vi "Gui_SetupExcitation.vi"(7 "Variant For Path":variant, 8 "error in (no error)":errorcluster, 10 "Excit Table Variant":variant, 11 "Variant":variant) -> (0 "error out":errorcluster caption="sortie d'erreur", 2 "Excit Table Variant Output":variant, 3 "Variant Output":variant)   [LabVIEW 2018]
doc: "This VI setup the parameters for the excitation waveforms.\n\n1. Init the table of Waveforms with the previous values.\n2. Wait for the user events, CTRL-Z is disabled.\n3. If any cell of the table has changed, start a Check and create a new excit script\n4. When OK is pushed, generate and store the waveforms to disk."
uses:
  controls/EXCIT_Form_Selector.ctl
  controls/EXPERT_Inputs.ctl
  controls/DIGIT_5122_Inputs.ctl
  <instrlib>/niScope/Controls/niScope trigger source.ctl
  controls/HSDIO_6541_Inputs.ctl
  <instrlib>/niHSDIO/niHSDIO.llb/niHSDIO_ctl Trigger Source Values (Ring).ctl
  controls/SOFTWARE_Inputs.ctl
  controls/AO_6711_Inputs.ctl
  controls/AWG_5421_Inputs.ctl
  <instrlib>/niFgen/niFgen.llb/niFgen_ctl Trigger Source Values (Ring).ctl
  controls/XML_Inputs.ctl
  controls/EXCIT_Table.ctl
  controls/SEQUENCE_Inputs.ctl
  controls/EXCIT_Inputs.ctl
  controls/DATA_Inputs.ctl
  controls/TIMING_Inputs.ctl
  controls/PROCESSING_Inputs.ctl
  controls/TRAPPING_Inputs.ctl
panel:
  in  "SEQUENCE Inputs":T1={"EXCIT Inputs"={"Number of Excitations"=1, "Script Text"="", "Table of Waveforms"=[]}, "DATA Inputs"={"Record Length"=524000, "Sample Rate"=2000000.0, "Data Type"=0, "Vertical Range"=10.0, "Acquisition Duration"=262.0}, "TIMING Inputs"={"Number of Acquisitions "=1, "Number of Accumulations"=1, "Table of Waveforms"=[], "Script Text"=""}, "PROCESSING Inputs"={"Reference Mass"=300.0939, "Cyclotron Freq"=255.727, "Magnetron Freq"=0.001}, "TRAPPING Inputs"={"Number of Channels"=4, "Init Values"=[2.0, 9.0, 2.0, 9.0], "Opening Values"=[0.0, 0.0, 0.0, 0.0], "Trapping Values"=[2.0, 9.0, 2.0, 9.0], "Emptying Values"=[-10.0, -10.0, -10.0, -10.0], "Adiabatic ON"=FALSE, "Adiabatic Duration"=100, "Adiabatic Waveforms"=["Adiabatic_None_2_2_2000", "Adiabatic_Ramp_9_0_2000", "Adiabatic_None_2_2_2000", "Adiabatic_RC_9_0_2000"], "Ions Refill ON"=FALSE, "Number of Ions Refills"=1, "Trapping Delay"=400.0, "Trapping Duration"=300.0}} {"TRAPPING Inputs"."Trapping Duration" min=2.0; "TRAPPING Inputs"."Trapping Delay" min=2.0; "TRAPPING Inputs"."Number of Ions Refills" min=1 max=1000; "TRAPPING Inputs"."Trapping Values" min=-10.0 max=10.0; "TRAPPING Inputs"."Init Values" min=-10.0 max=10.0; "TRAPPING Inputs"."Emptying Values" min=-10.0 max=10.0; "TRAPPING Inputs"."Opening Values" min=-10.0 max=10.0; "PROCESSING Inputs"."Magnetron Freq" format="%.5g"; "PROCESSING Inputs"."Cyclotron Freq" format="%.5g"; "PROCESSING Inputs"."Reference Mass" format="%.5g"; "TIMING Inputs"."Number of Accumulations" min=0 max=50 step=1; "TIMING Inputs"."Number of Acquisitions" min=1 max=10 step=1; "DATA Inputs"."Vertical Range" items=["0.2"=0.2, "0.4"=0.4, "1"=1.0, "2"=2.0, "4"=4.0, "10"=10.0]; "DATA Inputs"."Data Type" items=["I16", "DBL"]; "DATA Inputs"."Sample Rate" items=["1 MHz"=1000000.0, "2 MHz"=2000000.0, "5 MHz"=5000000.0, "10 MHz"=10000000.0, "20 MHz"=20000000.0, "25 MHz"=25000000.0, "50 MHz"=50000000.0, "100 MHz"=100000000.0]; "EXCIT Inputs"."Number of Excitations" min=1 max=10}
  in  "EXCIT Table":T7={"Number of Excits"=0, "Number of Ejects"=0, "Sampling Frequency"=0.0, "Waveforms Table"=[["Excit1", "name", "Swift", "0.5", "1200", "70", "150", "550", "0", "0", "0"]]}
  in  "EXPERT Inputs":T8={"DIGIT 5122 Inputs"={"Sample Rate"=1.0, "Resource Name"="Digitizer", "Channel Name"="0", "Trigger Source"="VAL_EXTERNAL", "Vertical Range"=10.0, "Trigger Level"=3.0}, "HSDIO 6541 Inputs"={"Resource Name"="SequencerHSDIO", "Clock Rate"=1000000.0, "Trigger Source"="PFI0"}, "SOFTWARE Inputs"={"Application Directory"=path "D:/S.O.F.T.S/LABVIEW/PIL", "Software Version"="1.0.0", "Data Path"=path "D:/PIRENEA/DATA", "XML Path"=path "D:/PIRENEA/DATA", "XML File Filter"="*.xml", "XML Saved Path"=path "D:/PIRENEA/DATA", "Excit Scripts Path"=path "D:/PIRENEA/EXCIT_SCRIPTS", "Excit Scripts File Filter"="*.txt", "Excit Waveforms Path"=path "D:/PIRENEA/EXCIT_WFMS", "Excit Waveforms File Filter"="*.bin", "Timing Scripts Path"=path "D:/PIRENEA/SEQUENCE_SCRIPTS", "Timing Scripts File Filter"="*.txt", "Timing Waveforms Path"=path "D:/PIRENEA/SEQUENCE_WFMS", "Timing Waveforms File Filter"="*.bin", "Trapping Waveforms Path"=path "D:/PIRENEA/TRAPPING_WFMS", "Trapping Waveforms File Filter"="*.bin"}, "AO 6711 Inputs"={"Physical Channels"="AnalogOutput/ao0:3", "Min Voltage"=-10.0, "Max Voltage"=10.0, "Trigger Source"="/AnalogOutput/PFI0", "Counter"="AnalogOutput/ctr0"}, "AWG 5421 Inputs"={"Resource Name"="WaveformGenerator", "Sample Rate"=0.0, "Trigger Type"=4, "Trigger Source"="PFI0", "Waveform Gain"=0.31, "Digital Filter ON"=TRUE}, "XML Inputs"={"Version Tag Name"="XML_Version", "Version String"="1.0"}} {"AWG 5421 Inputs"."Sample Rate" format="%.2p"; "AWG 5421 Inputs"."Trigger Type" items=["None", "Software Edge", "Digital Edge", "Digital Level"]; "AO 6711 Inputs"."Max Voltage" min=-10.0 max=10.0; "AO 6711 Inputs"."Min Voltage" min=-10.0 max=10.0; "HSDIO 6541 Inputs"."Clock Rate" format="%.2p"; "DIGIT 5122 Inputs"."Trigger Level" format="%.2f"; "DIGIT 5122 Inputs"."Vertical Range" format="%.2f"; "DIGIT 5122 Inputs"."Sample Rate" step=65535.0 format="%#_3p"}
  in  "CANCEL":bool
  in  "Sampling Frequency":dbl(ring)=10.0 caption="Sampling (MHz)" items=["10"=10.0, "20"=20.0, "25"=25.0, "50"=50.0, "100"=100.0]
  out "Excitation FFT":cluster{dbl[], "Power Spectrum (V^2 rms)":dbl[]}(graph)
  in  "Graph ID":i32
  out "Excitation Signal":T18(graph)
  in  "Excit Form":T19
  in  "CHECK":bool
  in  "Waveforms Table":i32(listbox)
  out "Number of Ejects":u16=1
  out "Number of Excits":u16=3
  out "Script Text":string
  in  "OK":bool
  # "GO_out"
  # "Gout"
  # "GI_in"
  # "Gin"
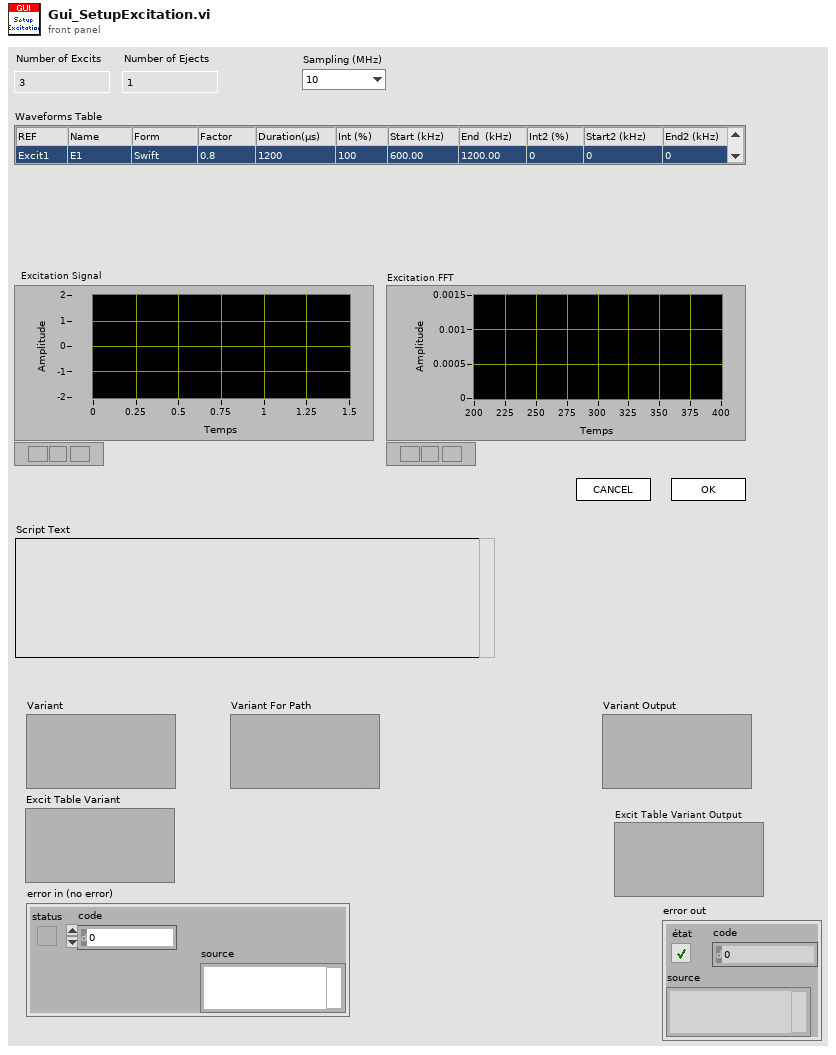
[diagram p1: front panel]
types:
  T1 = typedef "SEQUENCE_Inputs.ctl" = cluster{"EXCIT Inputs":T2, "DATA Inputs":T3, "TIMING Inputs":T4, "PROCESSING Inputs":T5, "TRAPPING Inputs":T6}
  T2 = typedef "EXCIT_Inputs.ctl" = cluster{"Number of Excitations":i32, "Script Text":string, "Table of Waveforms":string[]}
  T3 = typedef "DATA_Inputs.ctl" = cluster{"Record Length":i32, "Sample Rate":dbl, "Data Type":u8, "Vertical Range":dbl, "Acquisition Duration":dbl}
  T4 = typedef "TIMING_Inputs.ctl" = cluster{"Number of Acquisitions ":i16, "Number of Accumulations":i16, "Table of Waveforms":string[], "Script Text":string}
  T5 = typedef "PROCESSING_Inputs.ctl" = cluster{"Reference Mass":dbl, "Cyclotron Freq":dbl, "Magnetron Freq":dbl}
  T6 = typedef "TRAPPING_Inputs.ctl" = cluster{"Number of Channels":i32, "Init Values":dbl[], "Opening Values":dbl[], "Trapping Values":dbl[], "Emptying Values":dbl[], "Adiabatic ON":bool, "Adiabatic Duration":i32, "Adiabatic Waveforms":string[], "Ions Refill ON":bool, "Number of Ions Refills":i32, "Trapping Delay":dbl, "Trapping Duration":dbl}
  T7 = typedef "EXCIT_Table.ctl" = cluster{"Number of Excits":u16, "Number of Ejects":u16, "Sampling Frequency":dbl, "Waveforms Table":string[][]}
  T8 = typedef "EXPERT_Inputs.ctl" = cluster{"DIGIT 5122 Inputs":T9, "HSDIO 6541 Inputs":T11, "SOFTWARE Inputs":T13, "AO 6711 Inputs":T14, "AWG 5421 Inputs":T15, "XML Inputs":T17}
  T9 = typedef "DIGIT_5122_Inputs.ctl" = cluster{"Sample Rate":dbl, "Resource Name":refnum<k15>, "Channel Name":string, "Trigger Source":T10, "Vertical Range":dbl, "Trigger Level":dbl}
  T10 = typedef "niScope trigger source.ctl" = string
  T11 = typedef "HSDIO_6541_Inputs.ctl" = cluster{"Resource Name":refnum<k15>, "Clock Rate":dbl, "Trigger Source":T12}
  T12 = typedef "niHSDIO_ctl Trigger Source Values (Ring).ctl" = string
  T13 = typedef "SOFTWARE_Inputs.ctl" = cluster{"Application Directory":path, "Software Version":string, "Data Path":path, "XML Path":path, "XML File Filter":string, "XML Saved Path":path, "Excit Scripts Path":path, "Excit Scripts File Filter":string, "Excit Waveforms Path":path, "Excit Waveforms File Filter":string, "Timing Scripts Path":path, "Timing Scripts File Filter":string, "Timing Waveforms Path":path, "Timing Waveforms File Filter":string, "Trapping Waveforms Path":path, "Trapping Waveforms File Filter":string}
  T14 = typedef "AO_6711_Inputs.ctl" = cluster{"Physical Channels":tag, "Min Voltage":dbl, "Max Voltage":dbl, "Trigger Source":tag, "Counter":tag}
  T15 = typedef "AWG_5421_Inputs.ctl" = cluster{"Resource Name":refnum<k15>, "Sample Rate":dbl, "Trigger Type":u16, "Trigger Source":T16, "Waveform Gain":dbl, "Digital Filter ON":bool}
  T16 = typedef "niFgen_ctl Trigger Source Values (Ring).ctl" = string
  T17 = typedef "XML_Inputs.ctl" = cluster{"Version Tag Name":string, "Version String":string}
  T18 = cluster{"X Time":dbl[], "Signal Excitation":dbl[]}
  T19 = typedef "EXCIT_Form_Selector.ctl" = enum16{"Swift", "TwoSwift", "Chirp", "Sinus", "Ramp"}
  T20 = typedef "LVPoint32TypeDef.ctl" = cluster{"Horizontal":i32, "Vertical":i32}
  T21 = typedef "LVRowAndColumnTypeDef.ctl" = cluster{"Row":i32, "Column":i32}
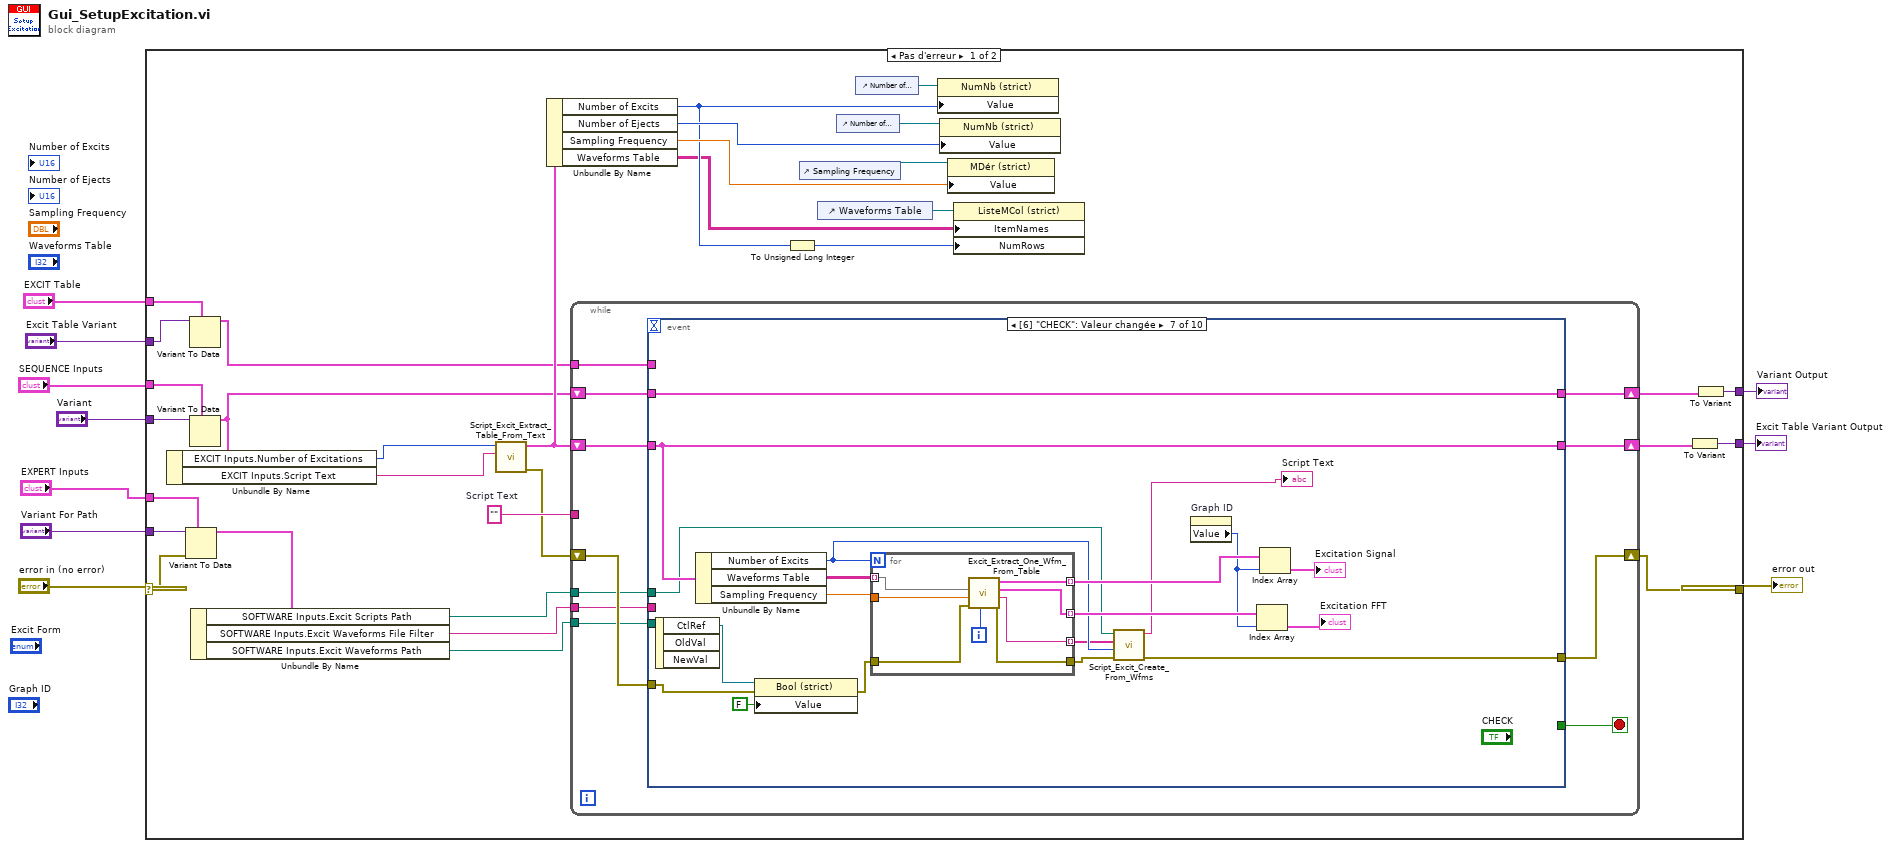
[diagram p0: block diagram]
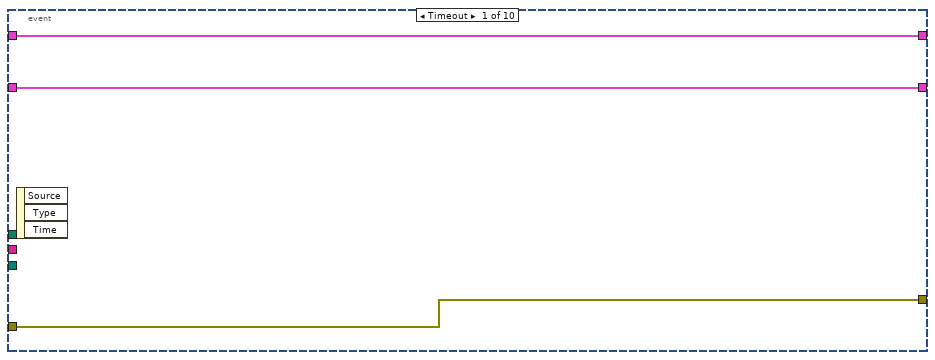
[diagram p2: hidden frame]
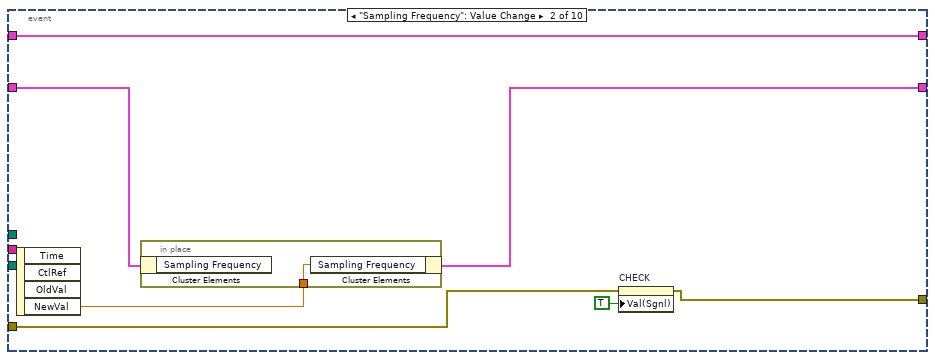
[diagram p3: hidden frame]
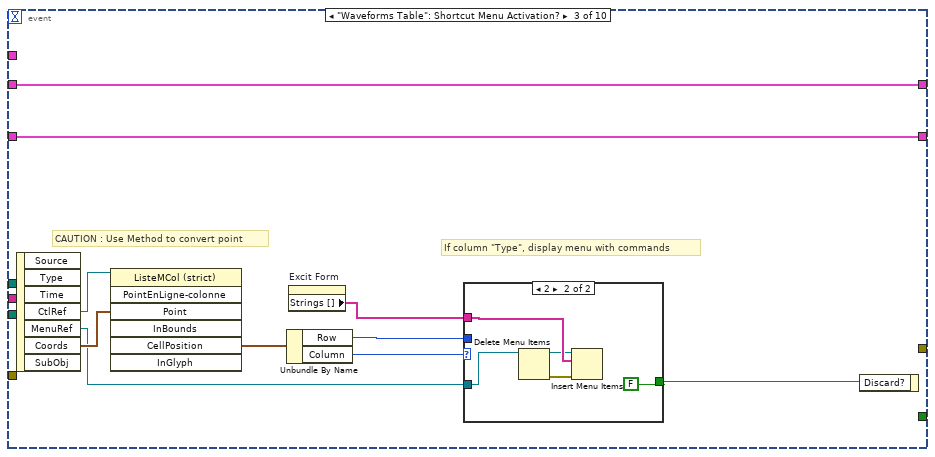
[diagram p4: hidden frame]
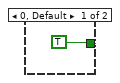
[diagram p5: hidden frame]
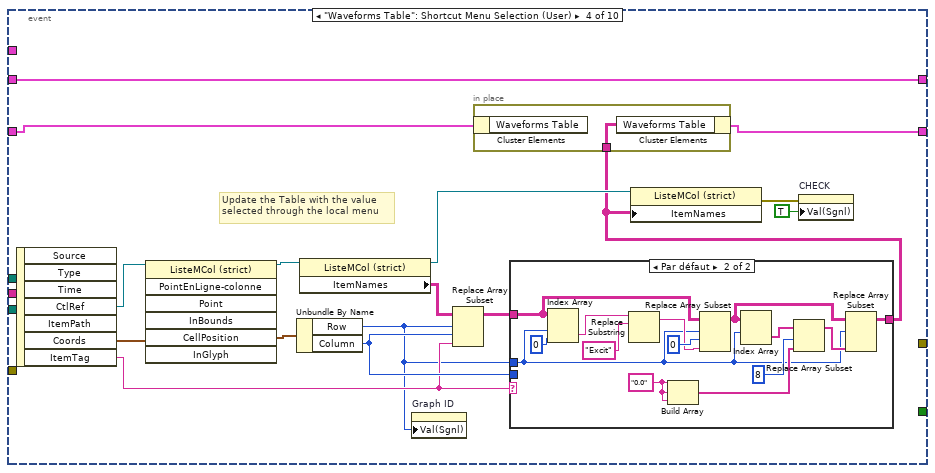
[diagram p6: hidden frame]
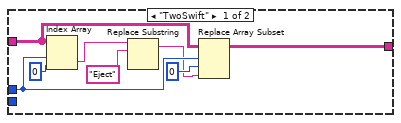
[diagram p7: hidden frame]
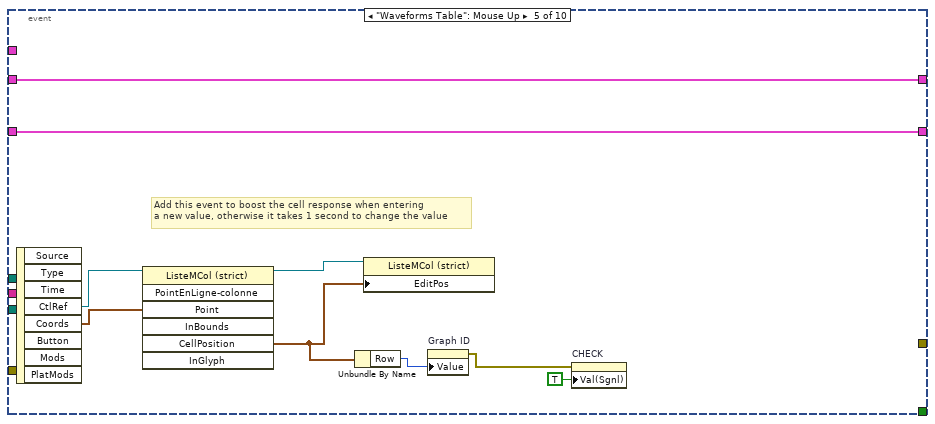
[diagram p8: hidden frame]
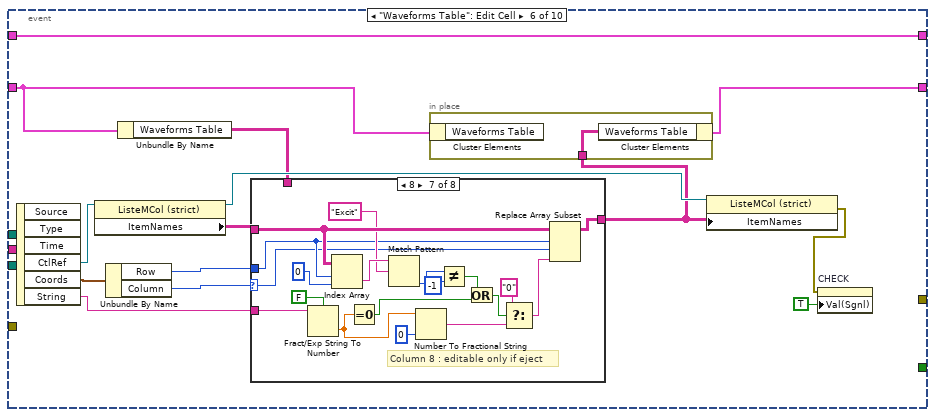
[diagram p9: hidden frame]
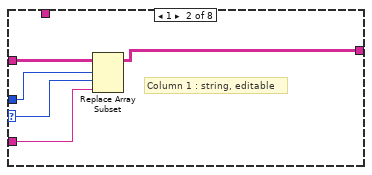
[diagram p11: hidden frame]
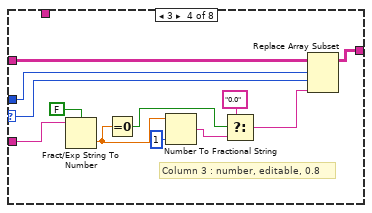
[diagram p13: hidden frame]
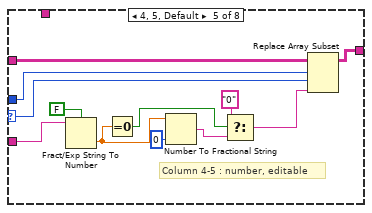
[diagram p14: hidden frame]
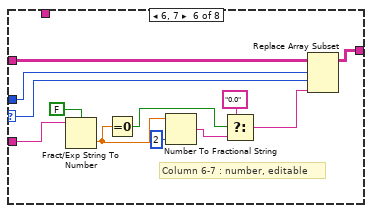
[diagram p15: hidden frame]
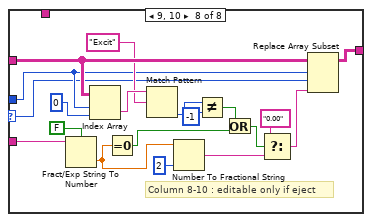
[diagram p16: hidden frame]
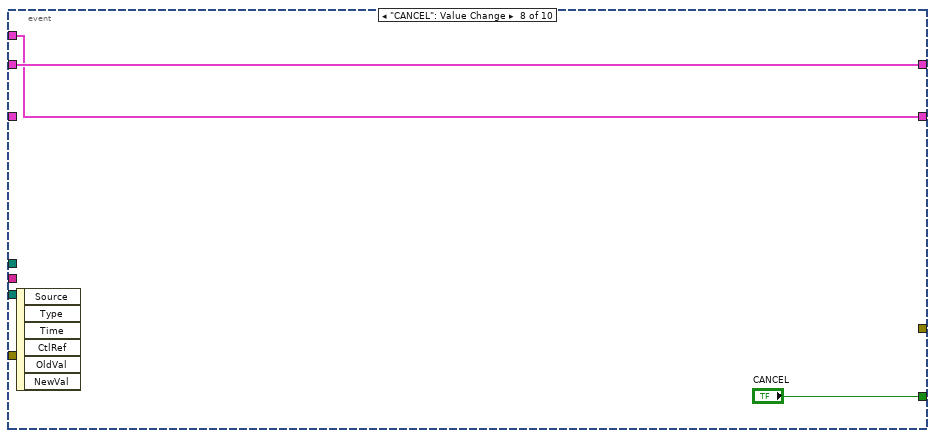
[diagram p17: hidden frame]
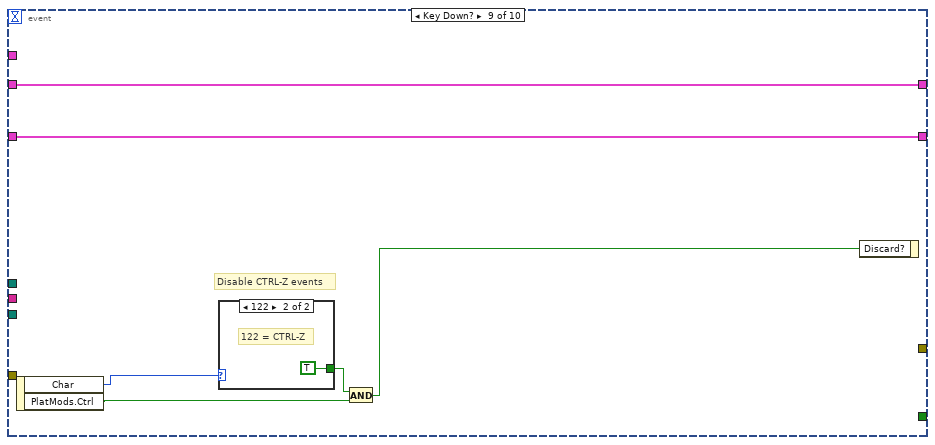
[diagram p18: hidden frame]
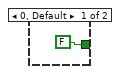
[diagram p19: hidden frame]
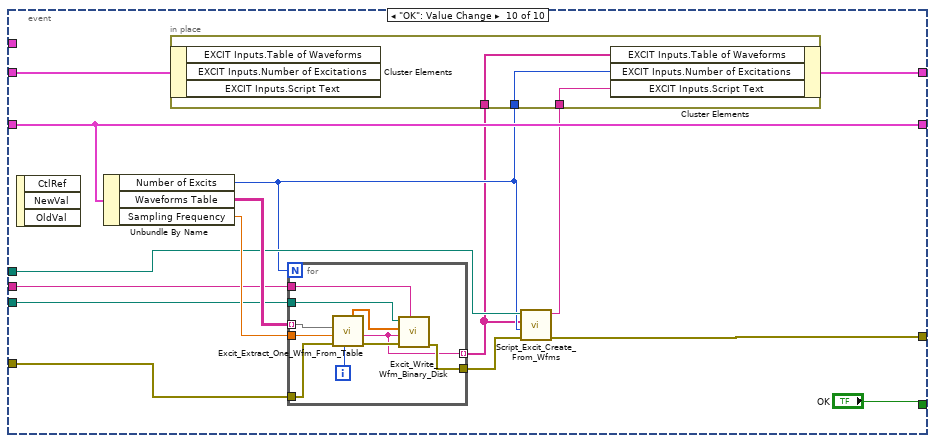
[diagram p20: hidden frame]
diagram:
  n1 = case shown="Pas d'erreur" "error in (no error)" {
    selector: "error in (no error)" -> [w38 w293]
    tunnel: [w26 w293] -> w9
    tunnel: "Variant" -> [w40 w292]
    tunnel: "Variant For Path" -> [w41 _]
    tunnel: [w39 w292] -> w6
    tunnel: [w17 w291] -> w4
    tunnel: "Excit Table Variant" -> [w16 w291]
    tunnel: "EXPERT Inputs" -> [w13 _]
    tunnel: "EXCIT Table" -> [w12 _]
    tunnel: "SEQUENCE Inputs" -> [w11 _]
    frame No Error {
      w31 = ""  # Script Text
      n2 = Variant To Data(error in=w38, type=w13, Variant=w41) -> (data=w42:T8)  [unwired: 1 out]
      n3 = Variant To Data(type=w12, Variant=w16) -> (data=w15:T7)  [unwired: 1 in, 1 out]
      n4 = Variant To Data(type=w11, Variant=w40) -> (data=w24:T1)  [unwired: 1 in, 1 out]
      n5 = Unbundle By Name(w24) -> ("EXCIT Inputs.Number of Excitations"=w14:i32, "EXCIT Inputs.Script Text"=w19:string)
      n6 = Unbundle By Name(w42) -> ("SOFTWARE Inputs.Excit Scripts Path"=w20:path, "SOFTWARE Inputs.Excit Waveforms File Filter"=w21:string, "SOFTWARE Inputs.Excit Waveforms Path"=w22:path)
      n7 = call "Script_Excit_Extract_Table_From_Text.vi"("Excit Text"=w19, "Number of Excitations"=w14) -> ("error out"=w27:errorcluster, "EXCIT Table"=w29:T7)  [unwired: 7 in, 1 out]
      n8 = Unbundle By Name(w29) -> ("Number of Excits"=w32:u16, "Number of Ejects"=w35:u16, "Sampling Frequency"=w34:dbl, "Waveforms Table"=w30:string[][])
      n9 = while {
        shift-right: [w49] -> w26
        shift-left: w27 -> [w53]
        shift-right: [w50] -> w18
        shift-left: w29 -> [w52]
        tunnel: w31 -> [_]
        shift-right: [w47] -> w25
        shift-left: w24 -> [w48]
        tunnel: w22 -> [w46]
        tunnel: w21 -> [w45]
        tunnel: w20 -> [w44]
        tunnel: w15 -> [w43]
        stop <- w51 stop-if-true
        n10 = event shown="[6] \"CHECK\": Valeur changée" {
          selector: _ -> [_ _ _ _ _ _ _ _ _ _]
          dyn-events: _ -> [_ _ _ _ _ _ _ _ _ _]
          timeout: _ -> [_ _ _ _ _ _ _ _ _ _]
          tunnel: w53 -> [w55 w57 _ _ _ _ w226 _ _ w273]
          tunnel: w52 -> [w56 w63 w67 w90 w126 w137 w243 _ w255 w274]
          tunnel: [w56 w61 w67 w89 w126 w133 w243 w252 w255 w274] -> w50
          tunnel: [_ _ _ _ _ _ _ "CANCEL" _ "OK"] -> w51
          tunnel: [w55 w58 _ _ _ _ w235 _ _ w266] -> w49
          tunnel: w48 -> [w54 w60 w65 w88 w125 w132 w234 w254 w260 w270]
          tunnel: [w54 w60 w65 w88 w125 w132 w234 w254 w260 w269] -> w47
          tunnel: w46 -> [_ _ _ _ _ _ _ _ _ w272]
          tunnel: w45 -> [_ _ _ _ _ _ _ _ _ w271]
          tunnel: w44 -> [_ _ _ _ _ _ w225 _ _ w267]
          tunnel: w43 -> [_ _ _ _ _ _ _ w252 _ _]
          event Timeout {
            n11 = event-data() -> ()  [unwired: 1 in, 3 out]
          }
          event "Sampling Frequency": Value Change {
            n12 = event-data() -> ("NewVal"=w62:dbl)  [unwired: 1 in, 3 out]
            n13 = in-place {
              in-place-border: w62 -> [w64]
              n14 = in-place-cluster #1(w63) -> ()  [unwired: 1 out]
              n15 = in-place-cluster #1("Sampling Frequency"=w64) -> (w61:T7)
            }
            n16 = property on="CHECK" class="Bool (strict)"(error in=w57, "Val(Sgnl)"=TRUE ("Valeur (Signalisation)")) -> (error out=w58:errorcluster)  [unwired: 1 in, 1 out]
          }
          event "Waveforms Table": Shortcut Menu Activation? {
            # "If column \"Type\", display menu with commands"
            # "CAUTION : Use Method to convert point"
            n17 = event-data() -> ("CtlRef"=w70:refnum<vi>, "MenuRef"=w69:refnum<k9>, "Coords"=w72:T20)  [unwired: 1 in, 4 out]
            n18 = invoke on="Nœud de méthode" class="ListeMCol (strict)" method="PointEnLigne-colonne"(reference=w70, "Point"=w72) -> ("CellPosition"=w71:T21)  [unwired: 5 in, 6 out]
            n19 = Unbundle By Name(w71) -> ("Row"=w73:i32, "Column"=w74:i32)
            n20 = property on="Excit Form" class="Énum (strict)"() -> ("Strings []"=w66:string[])  [unwired: 2 in, 2 out]
            n21 = case shown="2" w74 {
              tunnel: [TRUE FALSE] -> w68
              tunnel: w73 -> [_ _]
              tunnel: w66 -> [_ w79]
              tunnel: w69 -> [_ w76]
              frame 0, Default {
              }
              frame 2 {
                n22 = Delete Menu Items(9:w76) -> (0:w78:errorcluster, 3:w77:refnum<k9>)  [unwired: 3 in]
                n23 = Insert Menu Items(6:w78, 8:w79, 9:w77) -> ()  [unwired: 3 in, 3 out]
              }
            }
            n24 = event-data("Discard?"=w68) -> ()  [unwired: 1 in, 1 out]
          }
          event "Waveforms Table": Shortcut Menu Selection (User) {
            # "Update the Table with the value\nselected through the local menu"
            n25 = event-data() -> ("CtlRef"=w92:refnum<vi>, "Coords"=w91:T20, "ItemTag"=w85:string)  [unwired: 1 in, 4 out]
            n26 = invoke class="ListeMCol (strict)" method="PointEnLigne-colonne"(reference=w92, "Point"=w91) -> (reference out=w95:refnum<vi>, "CellPosition"=w96:T21)  [unwired: 5 in, 5 out]
            n27 = Unbundle By Name(w96) -> ("Row"=w84:i32, "Column"=w87:i32)
            n28 = property class="ListeMCol (strict)"(reference=w95) -> (reference out=w94:refnum<vi>, "ItemNames"=w93:string[][])  [unwired: 1 in, 1 out]
            n29 = property on="Graph ID" class="NumNb (strict)"("Val(Sgnl)"=w84) -> ()  [unwired: 2 in, 2 out]
            n30 = Replace Array Subset(array=w93, new element=w85, index (row)=w84, index (col)=w87) -> (w86:string[][])
            n31 = case shown="Par défaut" w85 {
              tunnel: w84 -> [w100 w106]
              tunnel: w87 -> [_ _]
              tunnel: w86 -> [w101 w115]
              tunnel: [w97 w105] -> w83
              frame "TwoSwift" {
                n32 = Index Array(array=w101, index (row)=w100, index (col)=0 ("indice désactivé (col)")) -> (element=w103:string)
                n33 = Replace Substring(4:"Eject" ("sous-chaîne (\"\")"), 5:w103) -> (1:w98:string)  [unwired: 2 in, 1 out]
                n34 = Replace Array Subset(array=w101, new element=w98, index (row)=w100, index (col)=0 ("indice désactivé (col)")) -> (w97:string[][])
              }
              frame Default {
                w112 = "0.0" ("nouvel élément/sous-tableau")
                n35 = Index Array(array=w115, index (row)=w106, index (col)=0 ("indice désactivé (col)")) -> (element=w117:string)
                n36 = Replace Substring(4:"Excit" ("sous-chaîne (\"\")"), 5:w117) -> (1:w113:string)  [unwired: 2 in, 1 out]
                n37 = Build Array(w112, w112, w112) -> (w111:string[])
                n38 = Replace Array Subset(array=w115, new element=w113, index (row)=w106, index (col)=0 ("indice désactivé (col)")) -> (w108:string[][])
                n39 = Index Array(array=w108, index (row)=w106) -> (element=w110:string[])  [unwired: 1 in]
                n40 = Replace Array Subset(array=w110, new element=w111, index=8 ("indice désactivé (col)")) -> (w107:string[])
                n41 = Replace Array Subset(array=w108, new element=w107, index (row)=w106) -> (w105:string[][])  [unwired: 1 in]
              }
            }
            n42 = in-place {
              in-place-border: w83 -> [w119]
              n43 = in-place-cluster #2(w90) -> ()  [unwired: 1 out]
              n44 = in-place-cluster #2("Waveforms Table"=w119) -> (w89:T7)
            }
            n45 = property class="ListeMCol (strict)"(reference=w94, "ItemNames"=w83) -> (error out=w82:errorcluster)  [unwired: 1 in, 1 out]
            n46 = property on="CHECK" class="Bool (strict)"(error in=w82, "Val(Sgnl)"=TRUE ("Valeur (Signalisation)")) -> ()  [unwired: 1 in, 2 out]
          }
          event "Waveforms Table": Mouse Up {
            # "Add this event to boost the cell response when entering\na new value, otherwise it takes 1 second to change the value"
            n47 = event-data() -> ("CtlRef"=w127:refnum<vi>, "Coords"=w124:T20)  [unwired: 1 in, 6 out]
            n48 = invoke class="ListeMCol (strict)" method="PointEnLigne-colonne"(reference=w127, "Point"=w124) -> (reference out=w128:refnum<vi>, "CellPosition"=w123:T21)  [unwired: 5 in, 5 out]
            n49 = Unbundle By Name(w123) -> ("Row"=w122:i32)
            n50 = property class="ListeMCol (strict)"(reference=w128, "EditPos"=w123) -> ()  [unwired: 1 in, 2 out]
            n51 = property on="Graph ID" class="NumNb (strict)"("Value"=w122) -> (error out=w121:errorcluster)  [unwired: 2 in, 1 out]
            n52 = property on="CHECK" class="Bool (strict)"(error in=w121, "Val(Sgnl)"=TRUE ("Valeur (Signalisation)")) -> ()  [unwired: 1 in, 2 out]
          }
          event "Waveforms Table": Edit Cell {
            n53 = event-data() -> ("CtlRef"=w134:refnum<vi>, "Coords"=w136:T21, "String"=w135:string)  [unwired: 1 in, 3 out]
            n54 = property class="ListeMCol (strict)"(reference=w134) -> (reference out=w140:refnum<vi>, "ItemNames"=w142:string[][])  [unwired: 1 in, 1 out]
            n55 = Unbundle By Name(w136) -> ("Row"=w131:i32, "Column"=w141:i32)
            n56 = Unbundle By Name(w137) -> ("Waveforms Table"=w139:string[][])
            n57 = case shown="8" w141 {
              selector: w141 -> [_ w145 _ w151 w163 w175 w187 w206]
              tunnel: w135 -> [_ w149 _ w162 w174 w186 w205 w224]
              tunnel: w142 -> [_ w147 _ w153 w165 w177 w197 w216]
              tunnel: w131 -> [_ w146 _ w152 w164 w176 w188 w207]
              tunnel: [w144 w148 w150 w161 w173 w185 w204 w223] -> w138
              tunnel: w139 -> [w144 _ w150 _ _ _ _ _]
              frame 0 {
                # "Column 0 : not editable"
              }
              frame 1 {
                # "Column 1 : string, editable"
                n58 = Replace Array Subset(array=w147, new element=w149, index (row)=w146, index (col)=w145) -> (w148:string[][])
              }
              frame 2 {
                # "Column 2 : choice into a menu"
              }
              frame 3 {
                # "Column 3 : number, editable, 0.8"
                n59 = Fract/Exp String To Number(use system decimal point (T)=FALSE ("utiliser le séparateur décimal du système (V)"), string=w162) -> (number=w157:dbl)  [unwired: 2 in, 1 out]
                n60 = Equal To 0?(x=w157) -> (x = 0?=w154:bool)
                n61 = Number To Fractional String(number=w157, precision (6)=i16 1 ("précision (6)")) -> (F-format string=w155:string)  [unwired: 2 in]
                n62 = Select(t="0.0", s=w154, f=w155) -> (s? t:f=w159:string)
                n63 = Replace Array Subset(array=w153, new element=w159, index (row)=w152, index (col)=w151) -> (w161:string[][])
              }
              frame 4, 5, Default {
                # "Column 4-5 : number, editable"
                n64 = Fract/Exp String To Number(use system decimal point (T)=FALSE ("utiliser le séparateur décimal du système (V)"), string=w174) -> (number=w169:dbl)  [unwired: 2 in, 1 out]
                n65 = Equal To 0?(x=w169) -> (x = 0?=w166:bool)
                n66 = Number To Fractional String(number=w169, precision (6)=i16 0 ("précision (6)")) -> (F-format string=w167:string)  [unwired: 2 in]
                n67 = Select(t="0", s=w166, f=w167) -> (s? t:f=w171:string)
                n68 = Replace Array Subset(array=w165, new element=w171, index (row)=w164, index (col)=w163) -> (w173:string[][])
              }
              frame 6, 7 {
                # "Column 6-7 : number, editable"
                n69 = Fract/Exp String To Number(use system decimal point (T)=FALSE ("utiliser le séparateur décimal du système (V)"), string=w186) -> (number=w181:dbl)  [unwired: 2 in, 1 out]
                n70 = Equal To 0?(x=w181) -> (x = 0?=w178:bool)
                n71 = Number To Fractional String(number=w181, precision (6)=i16 2 ("précision (6)")) -> (F-format string=w179:string)  [unwired: 2 in]
                n72 = Select(t="0.0", s=w178, f=w179) -> (s? t:f=w183:string)
                n73 = Replace Array Subset(array=w177, new element=w183, index (row)=w176, index (col)=w175) -> (w185:string[][])
              }
              frame 8 {
                # "Column 8 : editable only if eject"
                n74 = Fract/Exp String To Number(use system decimal point (T)=FALSE ("utiliser le séparateur décimal du système (V)"), string=w205) -> (number=w200:dbl)  [unwired: 2 in, 1 out]
                n75 = Index Array(array=w197, index (row)=w188, index (col)=0 ("indice désactivé (col)")) -> (element=w195:string)
                n76 = Equal To 0?(x=w200) -> (x = 0?=w192:bool)
                n77 = Match Pattern(string=w195, regular expression="Excit" ("expression régulière")) -> (offset past match=w191:i32)  [unwired: 1 in, 3 out]
                n78 = Number To Fractional String(number=w200, precision (6)=i16 0 ("précision (6)")) -> (F-format string=w198:string)  [unwired: 2 in]
                n79 = Not Equal?(x=w191, y=-1) -> (x != y?=w189:bool)
                n80 = Or(x=w189, y=w192) -> (x .or. y?=w193:bool)
                n81 = Select(t="0", s=w193, f=w198) -> (s? t:f=w202:string)
                n82 = Replace Array Subset(array=w197, new element=w202, index (row)=w188, index (col)=w187) -> (w204:string[][])
              }
              frame 9, 10 {
                # "Column 8-10 : editable only if eject"
                n83 = Fract/Exp String To Number(use system decimal point (T)=FALSE ("utiliser le séparateur décimal du système (V)"), string=w224) -> (number=w219:dbl)  [unwired: 2 in, 1 out]
                n84 = Index Array(array=w216, index (row)=w207, index (col)=0 ("indice désactivé (col)")) -> (element=w214:string)
                n85 = Equal To 0?(x=w219) -> (x = 0?=w211:bool)
                n86 = Match Pattern(string=w214, regular expression="Excit" ("expression régulière")) -> (offset past match=w210:i32)  [unwired: 1 in, 3 out]
                n87 = Number To Fractional String(number=w219, precision (6)=i16 2 ("précision (6)")) -> (F-format string=w217:string)  [unwired: 2 in]
                n88 = Not Equal?(x=w210, y=-1) -> (x != y?=w208:bool)
                n89 = Or(x=w208, y=w211) -> (x .or. y?=w212:bool)
                n90 = Select(t="0.00", s=w212, f=w217) -> (s? t:f=w221:string)
                n91 = Replace Array Subset(array=w216, new element=w221, index (row)=w207, index (col)=w206) -> (w223:string[][])
              }
            }
            n92 = in-place {
              in-place-border: w138 -> [w143]
              n93 = in-place-cluster #3(w137) -> ()  [unwired: 1 out]
              n94 = in-place-cluster #3("Waveforms Table"=w143) -> (w133:T7)
            }
            n95 = property class="ListeMCol (strict)"(reference=w140, "ItemNames"=w138) -> (error out=w130:errorcluster)  [unwired: 1 in, 1 out]
            n96 = property on="CHECK" class="Bool (strict)"(error in=w130, "Val(Sgnl)"=TRUE ("Valeur (Signalisation)")) -> ()  [unwired: 1 in, 2 out]
          }
          event "CHECK": Value Change {
            n97 = event-data() -> ("CtlRef"=w230:refnum<vi>)  [unwired: 1 in, 2 out]
            n98 = Unbundle By Name(w243) -> ("Number of Excits"=w233:u16, "Waveforms Table"=w242:string[][], "Sampling Frequency"=w241:dbl)
            n99 = property class="Bool (strict)"(reference=w230, error in=w226, "Value"=FALSE ("Valeur")) -> (error out=w228:errorcluster)  [unwired: 1 out]
            n100 = for {
              N: w233 -> [_]
              tunnel: w242 -> [w251] mode=indexing
              tunnel: w241 -> [w250]
              tunnel: [w248] -> w238 mode=indexing
              tunnel: [w247] -> w240 mode=indexing
              tunnel: [w246] -> w232 mode=indexing
              tunnel: w228 -> [w245]
              tunnel: [w244] -> w227
              i -> [w249]
              n101 = call "Excit_Extract_One_Wfm_From_Table.vi"("Excitation Number"=w249, "error in (no error)"=w245, "Sampling Frequency"=w250, "Waveforms Table"=w251) -> ("error out"=w244:errorcluster, "Waveform Name"=w246:string, "Excitation FFT"=w248:cluster{dbl[], "Power Spectrum (V^2 rms)":dbl[]}, "Excitation Signal"=w247:T18)  [unwired: 2 in, 2 out]
            }
            n102 = call "Script_Excit_Create_From_Wfms.vi"("error in (no error)"=w227, "Number of excitations"=w233, "Table of Waveforms"=w232, "Script Path"=w225) -> ("error out"=w235:errorcluster, "Script Text"=→"Script Text":string)  [unwired: 5 in, 1 out]
            n103 = property on="Graph ID" class="NumNb (strict)"() -> ("Value"=w237:i32)  [unwired: 2 in, 2 out]
            n104 = Index Array(array=w238, index=w237) -> (element=→"Excitation FFT":cluster{dbl[], "Power Spectrum (V^2 rms)":dbl[]})
            n105 = Index Array(array=w240, index=w237) -> (element=→"Excitation Signal":T18)
          }
          event "CANCEL": Value Change {
            n106 = event-data() -> ()  [unwired: 1 in, 6 out]
          }
          event Key Down? {
            # "Disable CTRL-Z events"
            n107 = event-data() -> ("Char"=w258:i16, "PlatMods.Ctrl"=w257:bool)  [unwired: 1 in]
            n108 = case shown="122" w258 {
              tunnel: [FALSE TRUE] -> w259
              frame 0, Default {
              }
              frame 122 {
                # "122 = CTRL-Z"
              }
            }
            n109 = And(x=w259, y=w257) -> (x .and. y?=w256:bool)
            n110 = event-data("Discard?"=w256) -> ()  [unwired: 1 in, 1 out]
          }
          event "OK": Value Change {
            n111 = event-data() -> ()  [unwired: 1 in, 3 out]
            n112 = Unbundle By Name(w274) -> ("Number of Excits"=w264:u16, "Waveforms Table"=w276:string[][], "Sampling Frequency"=w275:dbl)
            n113 = for {
              N: w264 -> [_]
              tunnel: w276 -> [w290] mode=indexing
              tunnel: w275 -> [w289]
              tunnel: w273 -> [w287]
              tunnel: w272 -> [w284]
              tunnel: w271 -> [w283]
              tunnel: [w282] -> w268
              tunnel: [w281] -> w263 mode=indexing
              i -> [w288]
              n114 = call "Excit_Extract_One_Wfm_From_Table.vi"("Excitation Number"=w288, "error in (no error)"=w287, "Sampling Frequency"=w289, "Waveforms Table"=w290) -> ("error out"=w286:errorcluster, "Waveform Name"=w281:string, "Signal Excitation"=w285:dbl[])  [unwired: 2 in, 3 out]
              n115 = call "Excit_Write_Wfm_Binary_Disk.vi"("Excit Waveforms File Filter"=w283, "error in (no error)"=w286, "Waveform Name"=w281, "Signal Excitation"=w285, "Excit Waveforms Path"=w284) -> ("error out"=w282:errorcluster)  [unwired: 6 in]
            }
            n116 = call "Script_Excit_Create_From_Wfms.vi"("error in (no error)"=w268, "Number of excitations"=w264, "Table of Waveforms"=w263, "Script Path"=w267) -> ("error out"=w266:errorcluster, "Script Text"=w265:string)  [unwired: 5 in, 1 out]
            n117 = in-place {
              in-place-border: w265 -> [w278]
              in-place-border: w264 -> [w279]
              in-place-border: w263 -> [w280]
              n118 = in-place-cluster #4(w270) -> ()  [unwired: 3 out]
              n119 = in-place-cluster #4("EXCIT Inputs.Table of Waveforms"=w280, "EXCIT Inputs.Number of Excitations"=w279, "EXCIT Inputs.Script Text"=w278) -> (w269:T1)
            }
          }
        }
      }
      n120 = To Unsigned Long Integer(number=w32) -> (unsigned 32bit integer=w28:u32)
      n121 = control-ref of="Sampling Frequency"() -> (w23:refnum<vi>)
      n122 = control-ref of="Waveforms Table"() -> (w33:refnum<vi>)
      n123 = control-ref of="Number of Ejects"() -> (w36:refnum<vi>)
      n124 = control-ref of="Number of Excits"() -> (w37:refnum<vi>)
      n125 = property class="NumNb (strict)"(reference=w37, "Value"=w32) -> ()  [unwired: 1 in, 2 out]
      n126 = property class="NumNb (strict)"(reference=w36, "Value"=w35) -> ()  [unwired: 1 in, 2 out]
      n127 = property class="MDér (strict)"(reference=w23, "Value"=w34) -> ()  [unwired: 1 in, 2 out]
      n128 = property class="ListeMCol (strict)"(reference=w33, "ItemNames"=w30, "NumRows"=w28) -> ()  [unwired: 1 in, 2 out]
      n129 = To Variant(anything=w18) -> (Variant=w17:variant)
      n130 = To Variant(anything=w25) -> (Variant=w39:variant)
    }
    frame Error {
    }
  }
  "error out" <- w9
  "Variant Output" <- w6
  "Excit Table Variant Output" <- w4
